vi "GetState.vi"(0 "Array Element":dbl, 1 "Array":dbl[](array[numeric]), 2 "dt":dbl, 5 "Loop Iteration":i32) -> (6 "Change State":bool, 7 "Rising/Falling Edge":bool, 8 "t":dbl)   [LabVIEW 2014]
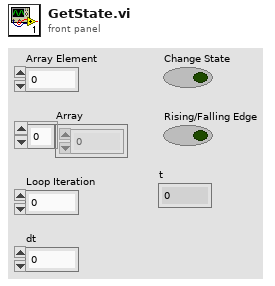
[diagram p1: front panel]
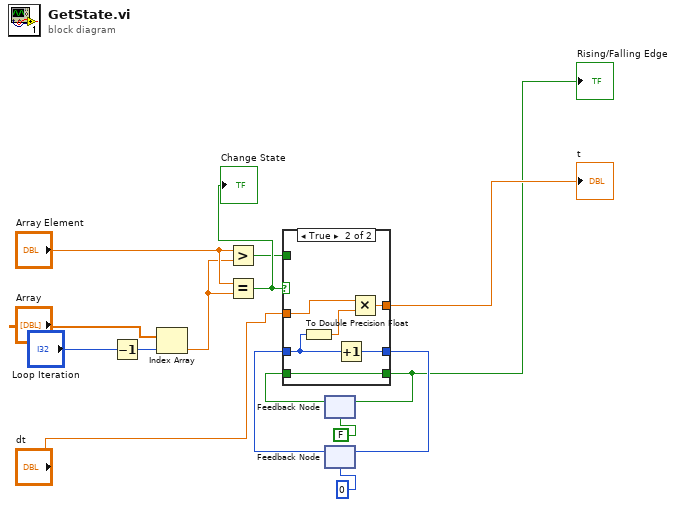
[diagram p0: block diagram]
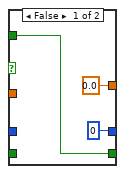
[diagram p2: hidden frame]
diagram:
  n1 = Decrement(x="Loop Iteration") -> (x-1=w2:i32)
  n2 = Index Array(array="Array", index=w2) -> (element=w4:dbl)
  n3 = Greater?(x="Array Element", y=w4) -> (0:w7:bool)
  n4 = Equal?(x="Array Element", y=w4) -> (x = y?=w15:bool)
  "Change State" <- w15
  n5 = feedback #1(FALSE) -> (w6:bool)
  n6 = feedback #2(0) -> (w12:i32)
  n7 = case shown="True" w15 {
    tunnel: w6 -> [_ w24]
    tunnel: [w18 w24] -> w8
    tunnel: w7 -> [w18 _]
    tunnel: [0 w19] -> w11
    tunnel: w12 -> [_ w20]
    tunnel: "dt" -> [_ w22]
    tunnel: [0.0 w21] -> w14
    frame False {
    }
    frame True {
      n8 = To Double Precision Float(number=w20) -> (double precision float=w23:dbl)
      n9 = Increment(x=w20) -> (x+1=w19:i32)
      n10 = Multiply(x=w22, y=w23) -> (x*y=w21:dbl)
    }
  }
  "t" <- w14
  "Rising/Falling Edge" <- w8
  n11 = feedback-in #1(w8) -> ()
  n12 = feedback-in #2(w11) -> ()
